vi "Obtain PES Connection.vi"(8 "Error In":errorcluster, 10 "port":u16, 11 "address":string) -> (0 "Error Out":errorcluster, 3 "TCP Out":refnum<k5>)   [LabVIEW 2016, in "OPI.lvclass"]
uses:
  OPI.lvclass
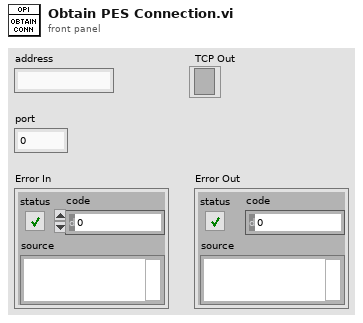
[diagram p1: front panel]
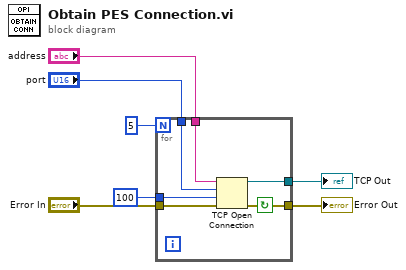
[diagram p0: block diagram]
diagram:
  n1 = for {
    N: 5 -> [_]
    tunnel: [w13] -> w2
    tunnel: "address" -> [w12]
    tunnel: "port" -> [w11]
    tunnel: "Error In" -> [w10]
    tunnel: [w9] -> w1
    tunnel: 100 ("timeout ms (60000)") -> [w8]
    stop <- w9 continue-if-true
    n2 = TCP Open Connection(address=w12, remote port or service name=w11, timeout ms (60000)=w8, error in (no error)=w10) -> (connection ID=w13:refnum<k5>, error out=w9:errorcluster)  [unwired: 1 in]
  }
  "TCP Out" <- w2
  "Error Out" <- w1
